vi "FTW-Actor.vi"(0 "FTW-TestExecutive-Core":refnum<class "FTW-TestExecutive-Core.lvclass">, 5 "FTW Actor Instance Configuration":string="{\n  \"Identity\": \"FTW Test Executive\",\n  \"InboxAddress\": \"inproc://ftwTestExec\",\n  \"LoggerAddress\": \"\",\n  \"Connections\": {},\n  \"Publishers\": {},\n  \"Subscriptions\": {},\n  \"Step Name Dictionary\": {},\n  \"Refresh Period\": 0.1\n}", 11 "ErrorIn":errorcluster) -> (15 "Error":errorcluster)   [LabVIEW 2015, in "FTW-TestExecutive-Core.lvclass"]
uses:
  FTW-TestExecutive-Core.lvclass
  FTW-TestExecutive-Core.lvclass/FTW-TestExecutive-Core.ctl
  FTW-TestExecutive-Core_State.ctl
  FTW-TestExecutive-Step-State.ctl
  Instance/FTW-ActorInstance.lvclass/FTW-ActorInstance.ctl
  JobSequencer/FTW-SEQ-Current.vi
  Message/Base/FTW-Message.lvclass
  Connector/FTW-ActorConnector.lvclass
  Instance/FTW-ActorInstance.lvclass
  Message/Request/FTW-Message-IncomingRequest.lvclass
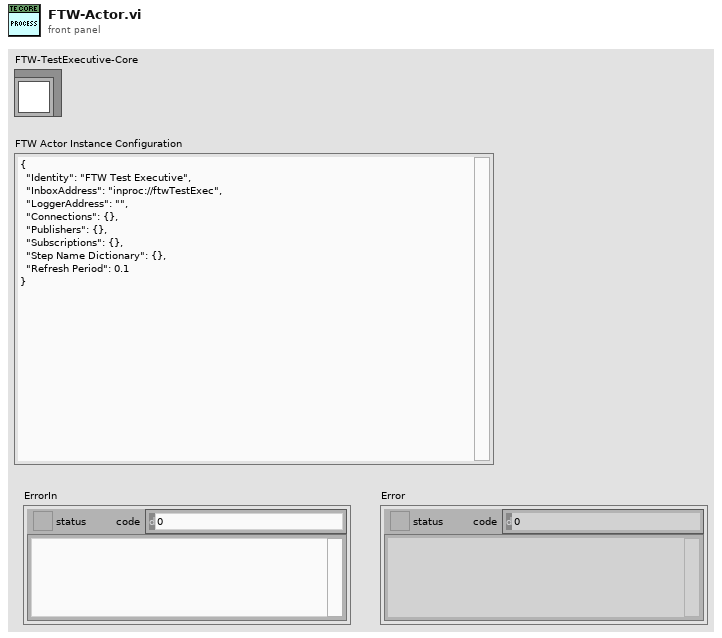
[diagram p1: front panel]
types:
  T1 = cluster{"Incoming Requests":refnum<event-registration>, "Local Messages":refnum<event-registration>, "Subscriber Registration":refnum<event-registration>}
  T2 = typedef "FTW-TestExecutive-Step-State.ctl" = enum8{"None", "Failed", "Passed", "Timed out", "Aborted"}
  T3 = typedef "FTW-TestExecutive-Core.lvclass/FTW-TestExecutive-Core_State.ctl" = enum8{"Unloaded", "Loaded", "Executing", "Paused"}
  T4 = typedef "FTW-TestExecutive-Step.ctl" = cluster{"Name":string, "Type":string, "Config":string, "Elapsed Time":dbl, "Passed":bool, "State":T2, "Results":T5}
  T5 = typedef "FTW-TestExecutive-Results.ctl" = cluster{"Start Time":timestamp, "Elapsed Time":dbl, "Passed":bool, "Additional Results":string}
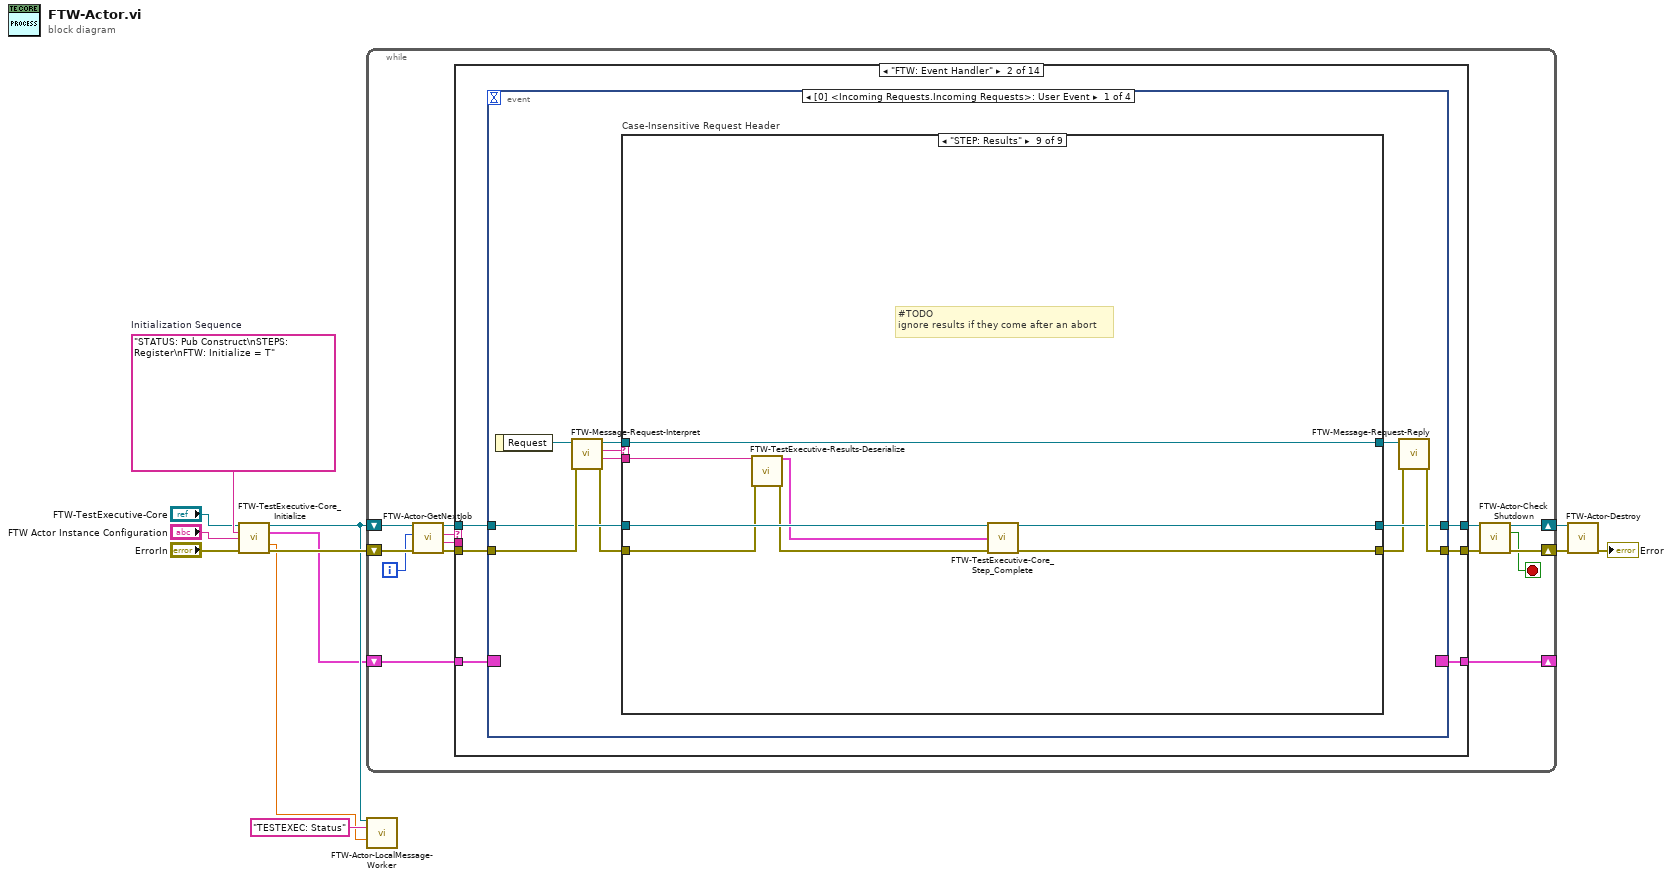
[diagram p0: block diagram]
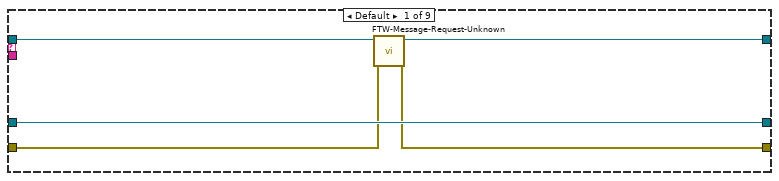
[diagram p3: hidden frame]
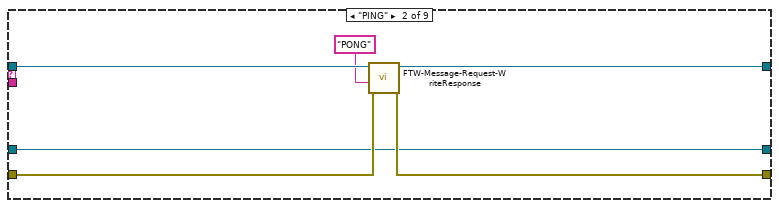
[diagram p4: hidden frame]
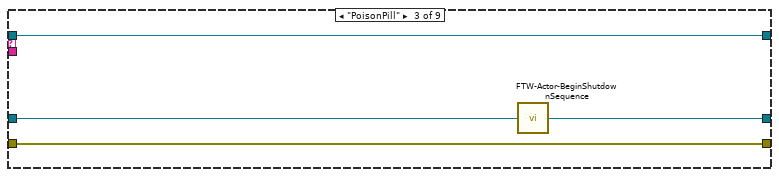
[diagram p5: hidden frame]
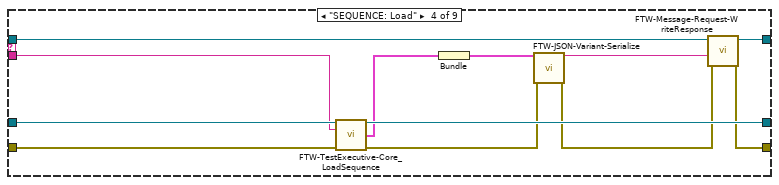
[diagram p6: hidden frame]
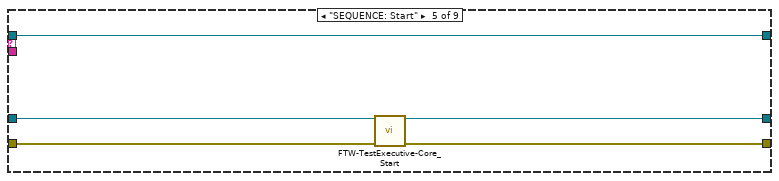
[diagram p7: hidden frame]
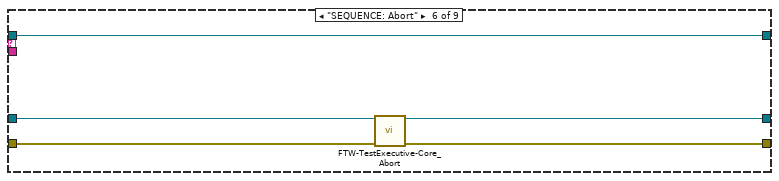
[diagram p8: hidden frame]
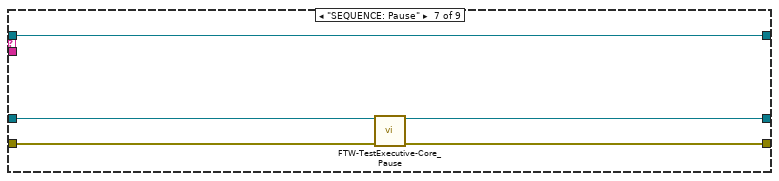
[diagram p9: hidden frame]
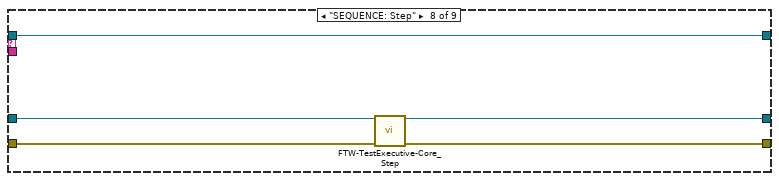
[diagram p10: hidden frame]
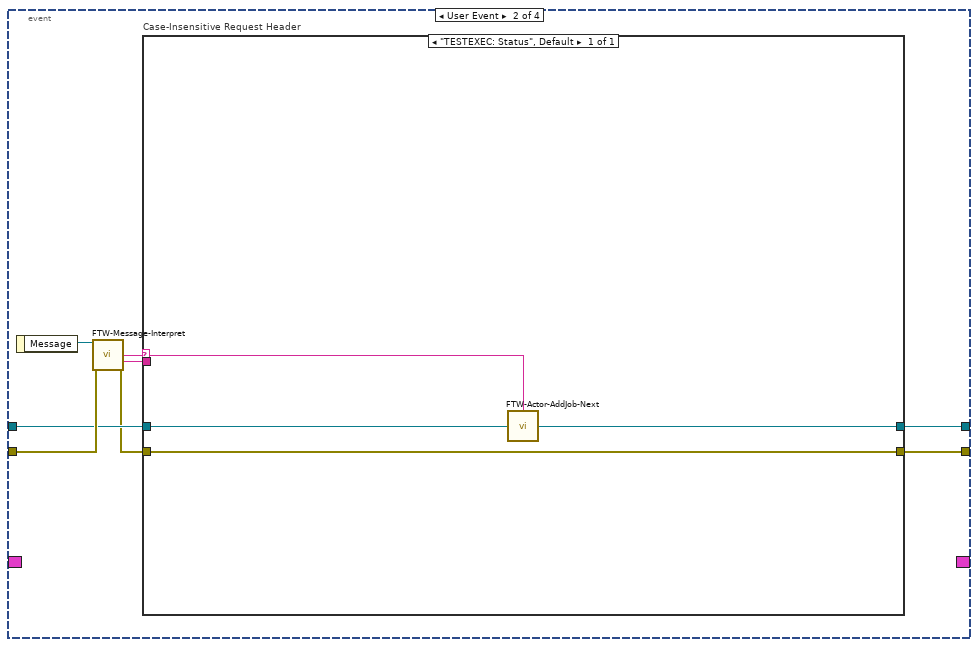
[diagram p11: hidden frame]
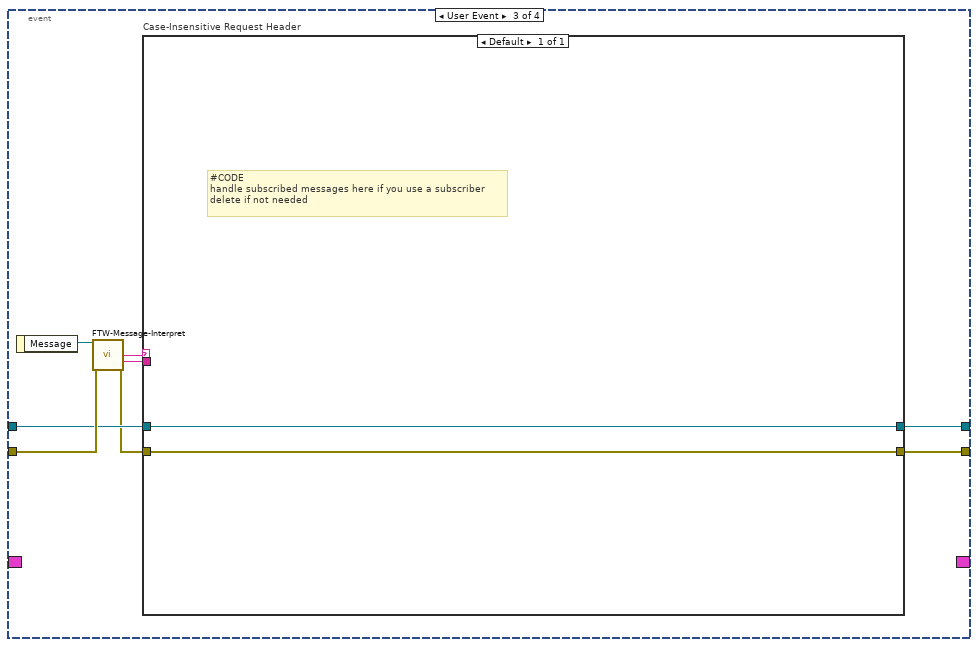
[diagram p12: hidden frame]
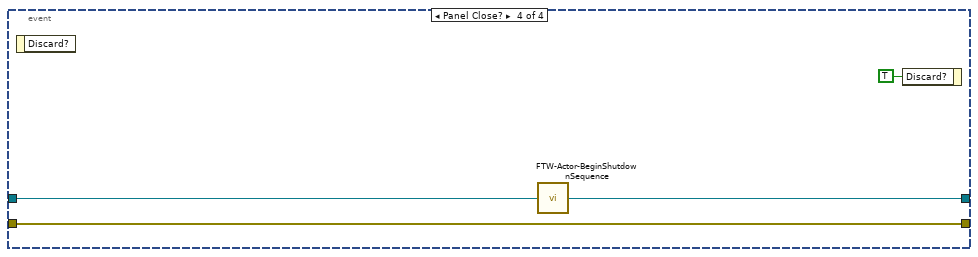
[diagram p13: hidden frame]
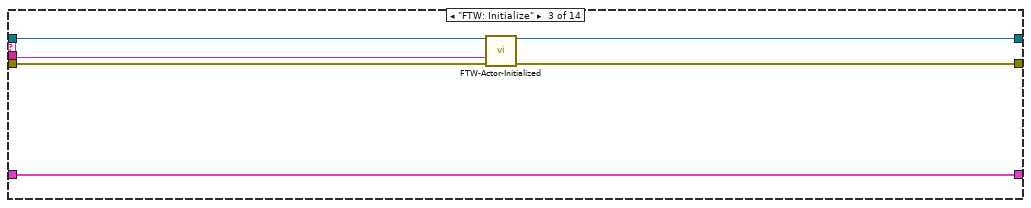
[diagram p14: hidden frame]
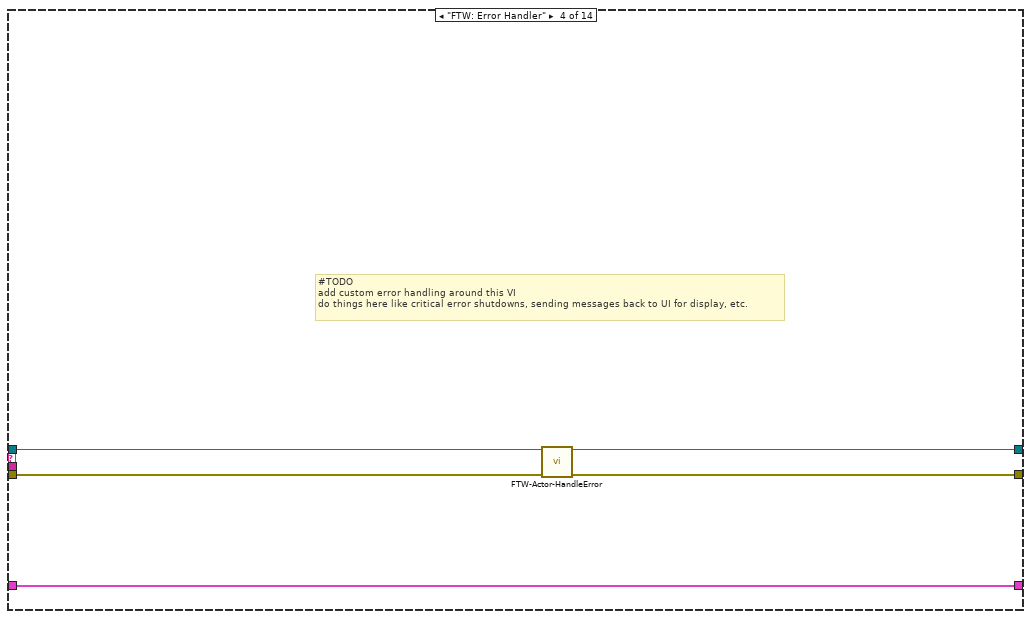
[diagram p15: hidden frame]
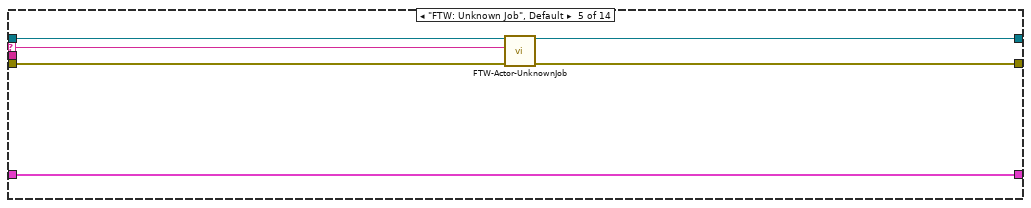
[diagram p16: hidden frame]
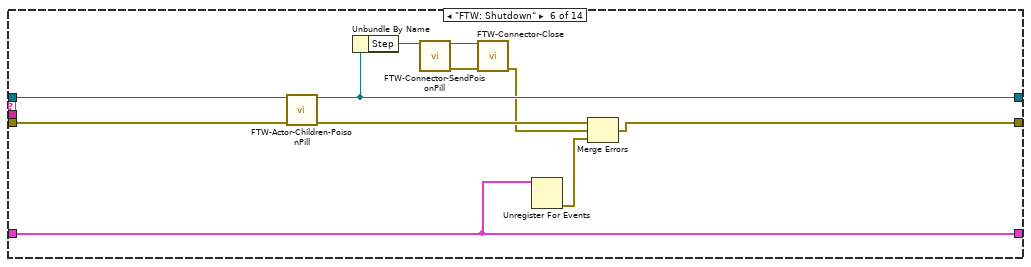
[diagram p17: hidden frame]
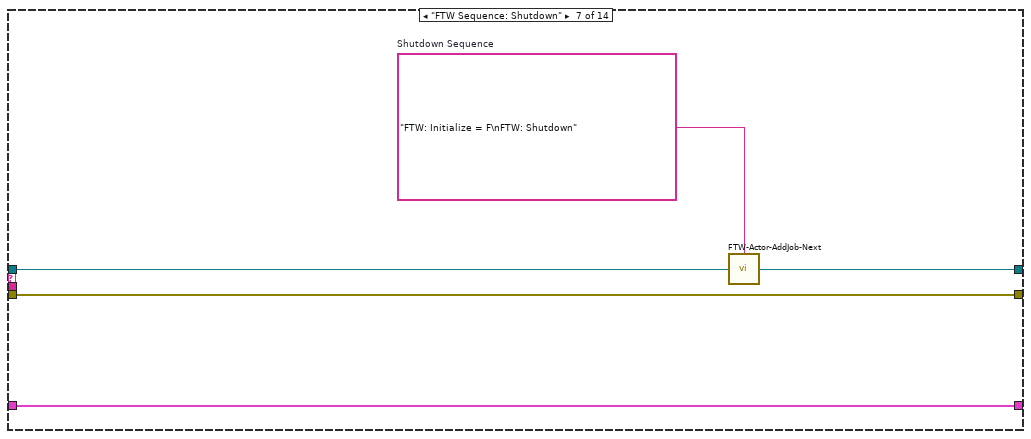
[diagram p18: hidden frame]
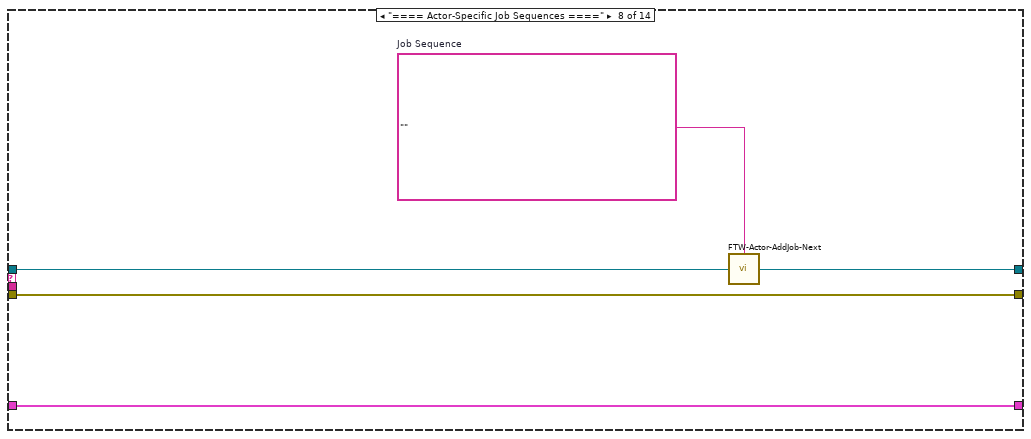
[diagram p19: hidden frame]
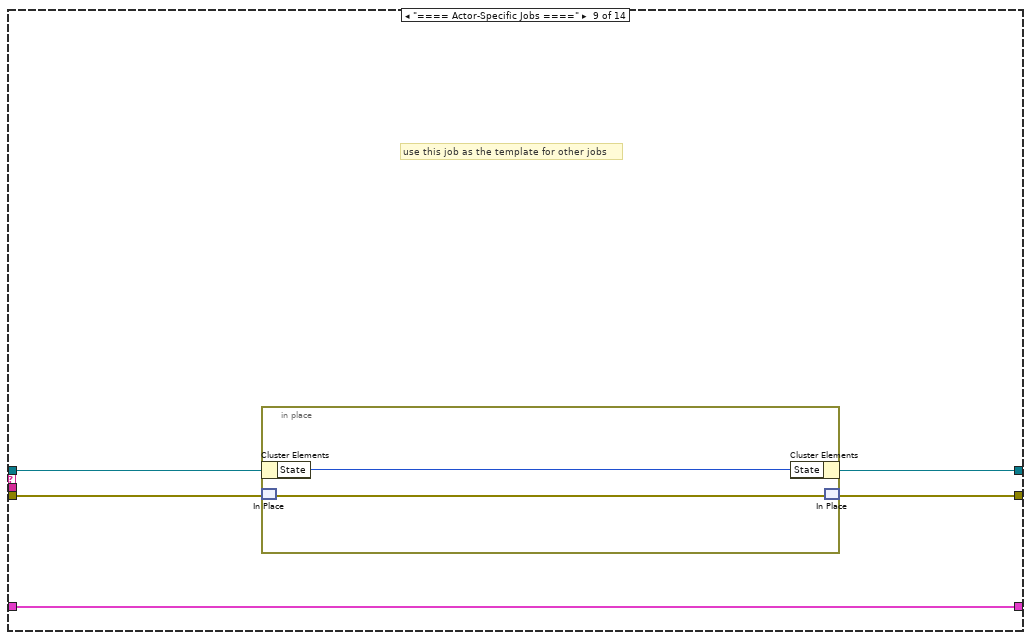
[diagram p20: hidden frame]
diagram:
  w2 = "STATUS: Pub Construct\nSTEPS: Register\nFTW: Initialize = T"  # Initialization Sequence
  n1 = call-dynamic "FTW-TestExecutive-Core_Initialize.vi"("Test Executive"="FTW-TestExecutive-Core", "Initialization Sequence"=w2, "FTW Actor Instance Configuration"="FTW Actor Instance Configuration", "error in (no error)"="ErrorIn") -> ("FTW-TestExecutive-Core Out"=w6:refnum<class "FTW-TestExecutive-Core.lvclass">, "Event Refnums"=w4:T1, "Refresh Period"=w5:dbl, "error out"=w9:errorcluster)  [unwired: 8 in]
  n2 = while {
    shift-right: [w16] -> w11
    shift-left: w9 -> [w23]
    shift-right: [w13] -> _
    shift-left: w4 -> [w26]
    shift-right: [w18] -> w12
    shift-left: w6 -> [w25]
    i -> [w14]
    stop <- w15 stop-if-true
    n3 = call "FTW-Actor-GetNextJob.vi"("error in"=w23, "Jobs Performed"=w14, "FTW Actor Instance"=w25) -> ("error out"=w22:errorcluster, "Job Data"=w20:string, "Job Name"=w21:string, "FTW Actor Instance out"=w24:refnum<class "FTW-TestExecutive-Core.lvclass">)  [unwired: 5 in]
    n4 = case shown="\"FTW: Event Handler\"" w21 {
      selector: w21 -> [_ _ _ _ w139 _ _ _ _ _ _ _ _ _]
      tunnel: [w28 w35 w130 w134 w142 w154 w159 w164 w168 w176 w206 w211 w216 w219] -> w17
      tunnel: w22 -> [w28 w34 w132 w136 w143 w155 w159 w164 w169 w175 w207 w212 w217 w225]
      tunnel: w26 -> [w29 w30 w133 w138 w144 w152 w160 w165 w170 w180 w208 w213 w218 w226]
      tunnel: [w29 w33 w133 w138 w144 w152 w160 w165 w170 w180 w208 w213 w218 w226] -> w13
      tunnel: w20 -> [_ _ w128 _ _ _ _ _ _ _ _ _ _ _]
      tunnel: [w27 w32 w131 w135 w140 w149 w157 w162 w166 w173 w205 w210 w215 w223] -> w19
      tunnel: w24 -> [w27 w31 w129 w137 w141 w150 w158 w163 w167 w174 w204 w209 w214 w224]
      frame "==== Featherweight Framework Jobs ====" {
      }
      frame "FTW: Event Handler" {
        n5 = event shown="[0] <Incoming Requests.Incoming Requests>: User Event" {
          selector: w30 -> [_ _ _ _]
          dyn-events: [_ _ _ _] -> w33
          timeout: _ -> [_ _ _ _]
          tunnel: [w45 w104 w116 w126] -> w35
          tunnel: w34 -> [w44 w108 w120 w126]
          tunnel: [w39 w105 w117 w124] -> w32
          tunnel: w31 -> [w43 w107 w119 w125]
          event User Event {
            n6 = event-data() -> ("Request"=w46:refnum<class "FTW-Message-IncomingRequest.lvclass">)  [unwired: 1 in]
            n7 = call "FTW-Message-Request-Interpret.vi"("error in"=w44, "FTW Incoming Request"=w46) -> ("error out"=w42:errorcluster, "Request Body"=w36:string, "Request Header"=w40:string, "FTW Incoming Request out"=w41:refnum<class "FTW-Message-IncomingRequest.lvclass">)  [unwired: 6 in]
            n8 = case "Case-Insensitive Request Header" shown="\"STEP: Results\"" w40 {
              tunnel: [w49 w55 w60 w64 w74 w79 w84 w89 w98] -> w38
              tunnel: w42 -> [w50 w56 w60 w70 w75 w80 w85 w90 w97]
              tunnel: [w51 w54 w61 w71 w76 w81 w86 w91 w99] -> w39
              tunnel: w43 -> [w51 w54 w59 w72 w77 w82 w87 w92 w100]
              tunnel: w41 -> [w48 w57 w58 w73 w78 w83 w88 w93 w101]
              tunnel: [w47 w53 w58 w68 w78 w83 w88 w93 w101] -> w37
              tunnel: w36 -> [_ _ _ w69 _ _ _ _ w94]
              frame Default {
                n9 = call "FTW-Message-Request-Unknown.vi"("error in"=w50, "FTW Incoming Request"=w48) -> ("error out"=w49:errorcluster, "FTW Incoming Request Out"=w47:refnum<class "FTW-Message-IncomingRequest.lvclass">)  [unwired: 8 in]
              }
              frame "PING" {
                n10 = call "FTW-Message-Request-WriteResponse.vi"("error in"=w56, "Response Body"="PONG" ("Response Header"), "FTW Incoming Request"=w57) -> ("error out"=w55:errorcluster, "FTW Incoming Request out"=w53:refnum<class "FTW-Message-IncomingRequest.lvclass">)  [unwired: 7 in]
              }
              frame "PoisonPill" {
                n11 = call "FTW-Actor-BeginShutdownSequence.vi"("FTW Actor Instance"=w59) -> ("FTW Actor Instance out"=w61:refnum<class "FTW-TestExecutive-Core.lvclass">)  [unwired: 3 in]
              }
              frame "SEQUENCE: Load" {
                n12 = call "FTW-TestExecutive-Core_LoadSequence.vi"("FTW-TestExecutive-Core In"=w72, "Sequence"=w69, "error in"=w70) -> ("FTW-TestExecutive-Core Out"=w71:refnum<class "FTW-TestExecutive-Core.lvclass">, "Loaded Sequence"=w62:T4[], "error out"=w67:errorcluster)  [unwired: 10 in]
                n13 = Bundle("Loaded Sequence"=w62) -> (w63:cluster{"Loaded Sequence":T4[]})  [unwired: 1 in]
                n14 = call "FTW-JSON-Variant-Serialize.vi"("Variant"=w63, "error in"=w67) -> ("JSON String"=w66:string, "error out"=w65:errorcluster)  [unwired: 12 in]
                n15 = call "FTW-Message-Request-WriteResponse.vi"("error in"=w65, "Response Body"=w66, "FTW Incoming Request"=w73) -> ("error out"=w64:errorcluster, "FTW Incoming Request out"=w68:refnum<class "FTW-Message-IncomingRequest.lvclass">)  [unwired: 7 in]
              }
              frame "SEQUENCE: Start" {
                n16 = call "FTW-TestExecutive-Core_Start.vi"("FTW-TestExecutive-Core In"=w77, "error in"=w75) -> ("FTW-TestExecutive-Core Out"=w76:refnum<class "FTW-TestExecutive-Core.lvclass">, "error out"=w74:errorcluster)  [unwired: 12 in]
              }
              frame "SEQUENCE: Abort" {
                n17 = call "FTW-TestExecutive-Core_Abort.vi"("FTW-TestExecutive-Core In"=w82, "error in"=w80) -> ("FTW-TestExecutive-Core Out"=w81:refnum<class "FTW-TestExecutive-Core.lvclass">, "error out"=w79:errorcluster)  [unwired: 12 in]
              }
              frame "SEQUENCE: Pause" {
                n18 = call "FTW-TestExecutive-Core_Pause.vi"("FTW-TestExecutive-Core In"=w87, "error in"=w85) -> ("FTW-TestExecutive-Core Out"=w86:refnum<class "FTW-TestExecutive-Core.lvclass">, "error out"=w84:errorcluster)  [unwired: 12 in]
              }
              frame "SEQUENCE: Step" {
                n19 = call "FTW-TestExecutive-Core_Step.vi"("FTW-TestExecutive-Core In"=w92, "error in"=w90) -> ("FTW-TestExecutive-Core Out"=w91:refnum<class "FTW-TestExecutive-Core.lvclass">, "error out"=w89:errorcluster)  [unwired: 12 in]
              }
              frame "STEP: Results" {
                # "#TODO\nignore results if they come after an abort"
                n20 = call "FTW-TestExecutive-Results-Deserialize.vi"("Serialized Results"=w94, "error in (no error)"=w97) -> ("Results"=w95:T5, "error out"=w96:errorcluster)  [unwired: 12 in]
                n21 = call "FTW-TestExecutive-Core_Step_Complete.vi"("FTW-TestExecutive-Core In"=w100, "Results"=w95, "error in"=w96) -> ("FTW-TestExecutive-Core Out"=w99:refnum<class "FTW-TestExecutive-Core.lvclass">, "error out"=w98:errorcluster)  [unwired: 11 in]
              }
            }
            n22 = call "FTW-Message-Request-Reply.vi"("FTW: Reply Error"=w38, "FTW Incoming Request"=w37) -> ("error out"=w45:errorcluster)  [unwired: 8 in, 1 out]
          }
          event User Event {
            n23 = event-data() -> ("Message"=w109:refnum<class "FTW-Message.lvclass">)  [unwired: 1 in]
            n24 = call-dynamic "FTW-Message-Interpret.vi"("FTW Message"=w109, "error in"=w108) -> ("Message Header"=w103:string, "Message Body"=w102:string, "error out"=w106:errorcluster)  [unwired: 9 in, 2 out]
            n25 = case "Case-Insensitive Request Header" shown="\"TESTEXEC: Status\", Default" w103 {
              selector: w103 -> [w110]
              tunnel: [w112] -> w104
              tunnel: w106 -> [w112]
              tunnel: [w111] -> w105
              tunnel: w107 -> [w113]
              tunnel: w102 -> [_]
              frame "TESTEXEC: Status", Default {
                n26 = call "FTW-Actor-AddJob-Next.vi"("Add Next in Job Queue"=w110, "FTW Actor Instance"=w113) -> ("FTW Actor Instance out"=w111:refnum<class "FTW-TestExecutive-Core.lvclass">)  [unwired: 2 in]
              }
            }
          }
          event User Event {
            n27 = event-data() -> ("Message"=w121:refnum<class "FTW-Message.lvclass">)  [unwired: 1 in]
            n28 = call-dynamic "FTW-Message-Interpret.vi"("FTW Message"=w121, "error in"=w120) -> ("Message Header"=w115:string, "Message Body"=w114:string, "error out"=w118:errorcluster)  [unwired: 9 in, 2 out]
            n29 = case "Case-Insensitive Request Header" shown="Default" w115 {
              tunnel: [w122] -> w116
              tunnel: w118 -> [w122]
              tunnel: [w123] -> w117
              tunnel: w119 -> [w123]
              tunnel: w114 -> [_]
              frame Default {
                # "#CODE\nhandle subscribed messages here if you use a subscriber\ndelete if not needed"
              }
            }
          }
          event Panel Close? {
            n30 = event-data() -> ()  [unwired: 1 in, 1 out]
            n31 = call "FTW-Actor-BeginShutdownSequence.vi"("FTW Actor Instance"=w125) -> ("FTW Actor Instance out"=w124:refnum<class "FTW-TestExecutive-Core.lvclass">)  [unwired: 3 in]
            n32 = event-data("Discard?"=TRUE) -> ()  [unwired: 1 in, 1 out]
          }
        }
      }
      frame "FTW: Initialize" {
        n33 = call-dynamic "FTW-Actor-Initialized.vi"("FTW Actor Instance"=w129, "Positive Init?"=w128, "error in"=w132) -> ("FTW Actor Instance out"=w131:refnum<class "FTW-TestExecutive-Core.lvclass">, "error out"=w130:errorcluster)  [unwired: 11 in]
      }
      frame "FTW: Error Handler" {
        # "#TODO\nadd custom error handling around this VI\ndo things here like critical error shutdowns, sending messages back to UI for display, etc."
        n34 = call-dynamic "FTW-Actor-HandleError.vi"("FTW Actor Instance"=w137, "error in"=w136) -> ("FTW Actor Instance out"=w135:refnum<class "FTW-TestExecutive-Core.lvclass">, "error out"=w134:errorcluster)  [unwired: 10 in, 2 out]
      }
      frame "FTW: Unknown Job", Default {
        n35 = call-dynamic "FTW-Actor-UnknownJob.vi"("FTW Actor Instance"=w141, "Unknown Job"=w139, "error in"=w143) -> ("FTW Actor Instance out"=w140:refnum<class "FTW-TestExecutive-Core.lvclass">, "error out"=w142:errorcluster)  [unwired: 11 in]
      }
      frame "FTW: Shutdown" {
        n36 = call "FTW-Actor-Children-PoisonPill.vi"("FTW-ActorInstance In"=w150, "error in"=w155) -> ("FTW-ActorInstance Out"=w149:refnum<class "FTW-TestExecutive-Core.lvclass">, "error out"=w151:errorcluster)  [unwired: 12 in]
        n37 = Unbundle By Name(w149) -> ("Step"=w148:refnum<class "FTW-ActorConnector.lvclass">)
        n38 = call-dynamic "FTW-Connector-SendPoisonPill.vi"("FTW Actor Connector"=w148) -> ("FTW Actor Connector out"=w147:refnum<class "FTW-ActorConnector.lvclass">, "error out"=w146:errorcluster)  [unwired: 9 in, 4 out]
        n39 = call-dynamic "FTW-Connector-Close.vi"("FTW Actor Connector"=w147, "error in"=w146) -> ("error out"=w145:errorcluster)  [unwired: 13 in]
        n40 = Unregister For Events(event registration refnum=w152) -> (error out=w153:errorcluster)  [unwired: 1 in]
        n41 = Merge Errors(w151, w145, w153) -> (w154:errorcluster)
      }
      frame "FTW Sequence: Shutdown" {
        w156 = "FTW: Initialize = F\nFTW: Shutdown"  # Shutdown Sequence
        n42 = call "FTW-Actor-AddJob-Next.vi"("Add Next in Job Queue"=w156, "FTW Actor Instance"=w158) -> ("FTW Actor Instance out"=w157:refnum<class "FTW-TestExecutive-Core.lvclass">)  [unwired: 2 in]
      }
      frame "==== Actor-Specific Job Sequences ====" {
        w161 = ""  # Job Sequence
        n43 = call "FTW-Actor-AddJob-Next.vi"("Add Next in Job Queue"=w161, "FTW Actor Instance"=w163) -> ("FTW Actor Instance out"=w162:refnum<class "FTW-TestExecutive-Core.lvclass">)  [unwired: 2 in]
      }
      frame "==== Actor-Specific Jobs ====" {
        # "use this job as the template for other jobs"
        n44 = in-place {
          n45 = in-place-cluster #1(w167) -> ("State"=w171:T3)
          n46 = in-place-match #2(w169) -> (w172:errorcluster)
          n47 = in-place-cluster #1("State"=w171) -> (w166:refnum<class "FTW-TestExecutive-Core.lvclass">)
          n48 = in-place-match #2(w172) -> (w168:errorcluster)
        }
      }
      frame "TESTEXEC: Status" {
        n49 = Unbundle By Name(w174) -> ("State"=w178:T3, "Step Start Time"=w179:dbl, "Step Timeout"=w177:dbl)
        n50 = case shown="\"Executing\"" w178 {
          tunnel: w179 -> [_ w190 _]
          tunnel: w177 -> [_ w188 _]
          tunnel: [w181 w185 w200] -> w176
          tunnel: w175 -> [w181 w187 w200]
          tunnel: w174 -> [w182 w184 w201]
          tunnel: [w182 w186 w201] -> w173
          frame "Unloaded", "Loaded" {
          }
          frame "Executing" {
            n51 = call "FTW-Time-Uptime.vi"("Previous Uptime"=w190) -> ("Elapsed Time"=w189:dbl)  [unwired: 12 in, 2 out]
            n52 = Greater?(x=w189, y=w188) -> (0:w183:bool)
            n53 = case shown="True" w183 {
              tunnel: w187 -> [w191 w199]
              tunnel: [w192 w198] -> w186
              tunnel: [w191 w196] -> w185
              tunnel: w184 -> [w192 w195]
              frame False {
              }
              frame True {
                n54 = call "FTW-TestExecutive-Core_Step_SetStatus.vi"("FTW-TestExecutive-Core In"=w195, "State"=FTW-TestExecutive-Step-State."Timed out", "error in"=w199) -> ("FTW-TestExecutive-Core Out"=w194:refnum<class "FTW-TestExecutive-Core.lvclass">, "error out"=w196:errorcluster)  [unwired: 11 in]
                n55 = Bundle By Name(cluster=w194, "State"=FTW-TestExecutive-Core_State."Loaded") -> (w198:refnum<class "FTW-TestExecutive-Core.lvclass">)
              }
            }
          }
          frame "Paused" {
          }
        }
      }
      frame "STATUS: Pub Construct" {
        # "add status publisher for test exec"
        n56 = call "FTW-Actor-Publisher-Add.vi"("FTW-ActorInstance In"=w204, "Publisher Name"="TestExecStatusPub", "Publisher URI"="inproc://*", "error in"=w207) -> ("FTW-ActorInstance Out"=w205:refnum<class "FTW-TestExecutive-Core.lvclass">, "error out"=w206:errorcluster)  [unwired: 10 in]
      }
      frame "STEPS: Register" {
        n57 = call-dynamic "FTW-TestExecutive-Core_StepTypes_Define.vi"("FTW-TestExecutive-Core In"=w209, "error in"=w212) -> ("FTW-TestExecutive-Core Out"=w210:refnum<class "FTW-TestExecutive-Core.lvclass">, "error out"=w211:errorcluster)  [unwired: 12 in]
      }
      frame "STEP: Execute" {
        n58 = call "FTW-TestExecutive-Core_Step_Launch.vi"("FTW-TestExecutive-Core In"=w214, "error in"=w217) -> ("FTW-TestExecutive-Core Out"=w215:refnum<class "FTW-TestExecutive-Core.lvclass">, "error out"=w216:errorcluster)  [unwired: 12 in]
      }
      frame "CONN: Ask" {
        # "example of asking a connected actor something\n\nuse the connection to call the actor API"
        n59 = call "FTW-Actor-Connection-Get.vi"("FTW-ActorInstance In"=w224, "Connector Name"="ConnectionOne" ("Publisher Name"), "error in"=w225) -> ("FTW-ActorInstance Out"=w223:refnum<class "FTW-TestExecutive-Core.lvclass">, "FTW Actor Connector"=w221:refnum<class "FTW-ActorConnector.lvclass">, "error out"=w220:errorcluster)  [unwired: 10 in]
        n60 = flat-sequence {
          tunnel: w221 -> [_]
          tunnel: w220 -> [w227]
          tunnel: [w227] -> w219
          frame #0 {
          }
        }
      }
    }
    n61 = call "FTW-Actor-CheckShutdown.vi"("FTW Actor Instance"=w19, "error in"=w17) -> ("FTW Actor Instance out"=w18:refnum<class "FTW-TestExecutive-Core.lvclass">, "Shutdown?"=w15:bool, "error out"=w16:errorcluster)  [unwired: 11 in]
  }
  n62 = call "FTW-Actor-LocalMessage-Worker.vi"("FTW-ActorInstance In"=w6, "Message Header"="TESTEXEC: Status", "Send Rate"=w5) -> ()  [unwired: 13 in]
  n63 = call-dynamic "FTW-Actor-Destroy.vi"("FTW Actor Instance"=w12, "error in"=w11) -> ("error out"=→"Error":errorcluster)  [unwired: 13 in]
